vi "impulse.vi"() -> ()   [LabVIEW 2015]
uses:
  <vilib>/express/express analysis/Spectral/Block/exnSpectralBlock spectral measurements RMS poly.vi
  <vilib>/express/express analysis/Spectral/Block/exnSpectralBlock spectral measurements RMS WFM.vi
  <vilib>/express/express analysis/Spectral/XNode/ExpressSpectralMeasurementsBlockNode.xnode
panel:
  out "error out":errorcluster
  in  "error in":errorcluster
  in  "Stop Button":bool
  in  "Rate":dbl=4000.0
  in  "Averages":dbl=10.0
  in  "Time (sec)":dbl=0.2
  out "FFT":cluster{"f0":dbl, "df":dbl, "magnitude":dbl[]}(graph)={"f0"=0.0, "df"=5.0, "magnitude"=[-76.96384322517771, -76.42679486233023, -72.85666642341076, -71.38647319065812, -70.14662433053286, -67.52954782473027, -68.48400168826473, -72.39914045035815, -73.87927581141093, -76.83283155880913, -68.18744880683296, -68.4682142733081, -65.23066848529315, -69.27070672338077, -71.0175747468924, -73.06274814845091, -70.13008167063762, -76.36995304006233, -75.77281317706263, -75.55570327595308, -69.78822078992803, -68.74398541895071, -71.8694071583193, -64.49841394636594, -62.6804616224581, -66.92788976349084, -61.60831729458516, -62.28071166288875, -57.653094015959745, -53.22277642336562, -45.26642983314452, -34.38407325316543, -29.142428384242063, -32.91095376852357, -44.25910915056805, -53.18033994048258, -59.4769321245915, -61.072306867585986, -67.42925441188714, -66.84917435783197, -68.66575018363679, -69.7591404271292, -71.03152031159054, -70.9893803258124, -68.38199207817071, -72.00448948746491, -68.01256152070326, -67.9316604541294, -68.08904411886591, -67.99455524325555, -68.45174479754071, -67.30715293001177, -69.20448006996517, -67.5542171673227, -70.46036907543153, -67.58462190001059, -70.28521679448141, -68.2887848064451, -71.01143222397984, -67.6571419445792, -64.8548009674459, -63.820552592220196, -59.22957694885139, -52.5909165554164, -45.60812098925769, -42.002043104158304, -43.1903623164439, -49.22576249781181, -54.3780871023297, -57.86663523243824, -61.37809785909429, -65.05174356042342, -64.63930926360648, -64.11899085358468, -66.2159413011727, -68.93297817441363, -67.65564424572169, -72.9860971642846, -70.8799512804249, -74.08075178434568, -73.53297038665296, -74.1334014855353, -73.62832977107102, -74.71414022509782, -69.6031859659534, -70.21674262130918, -70.17200512340543, -68.8508491485637, -67.28457145151319, -67.18061516068467, -65.54873963096921, -65.0729025484959, -64.35822791542905, -61.6748482258688, -61.782563080853635, -63.04528441289746, -58.154907346835685, -54.71707233923819, -52.32393128109371, -53.81718862378017, -56.7098876504202, -62.68891050590184, -66.62682561685475, -66.83733759788919, -71.2450353090801, -65.65204670851749, -65.17581139718769, -68.16827380079054, -67.40143134206475, -67.11770285587087, -70.19719870933834, -67.87984510416211, -68.79990506319385, -71.59294042822327, -70.91779533548043, -71.37930707684605, -73.18467103419579, -74.5011236027276, -76.60216907463567, -76.36296374745734, -76.45992372880559, -73.34261139404917, -77.95153696406045, -72.05050193571411, -71.29187913220059, -69.62859338533406, -64.40675607726061, -63.35442870012269, -61.72236714640202, -57.662771066358744, -52.796942960053, -46.34620361215351, -42.96197942024599, -45.17513798727579, -51.64747739619454, -58.029749238153265, -63.58841604408845, -70.76172686722498, -74.0431297812586, -74.9889309405747, -72.52553568570184, -79.44586305416209, -75.57818400702382, -80.6207143763097, -75.45228631067108, -74.26272136812842, -77.05517432462732, -80.75333514371572, -74.95436340173164, -77.7343141563188, -75.08345145489872, -73.34506006774251, -77.47698539624334, -81.19713534940053, -76.00473310433264, -75.42901615687343, -78.20571496514997, -86.39258933247719, -79.06551886154028, -77.89189547590172, -76.14393205620179, -72.93536567376772, -67.13766563289994, -60.84765888264903, -51.58315520325594, -46.47566832056483, -48.54804136630699, -56.46988012444743, -64.11642116158627, -64.5786281646024, -68.2789885346105, -75.50097459432686, -71.83221105685784, -83.66782491984347, -75.27823026551795, -79.91546413793313, -84.70037150416685, -80.37298184889379, -90.1157689151875, -79.92871393538528, -84.83378559249539, -90.65780463744412, -81.34788679276531, -81.13427799763167, -86.04606910008829, -86.06641360780303, -78.28991024552357, -89.64816068193657, -80.8415647684923, -76.86141990488758, -83.5463763501563, -82.65373729606111, -73.75131007003918, -73.1974150846216, -73.1389997357267, -71.88763088714863, -68.92135534739391, -60.2018529106938, -55.89209342955029, -59.20342116383752, -66.40916834876512, -72.63324321776088, -75.30892178225696, -85.14599467373729, -82.6371796990402, -76.8616932072628, -78.73131182614961, -77.60434868224353, -78.05227652249873, -83.70865742856554, -82.55297700984232, -94.03545009272696, -80.044471309499, -81.33544305439534, -87.20188454329838, -98.67608701021186, -81.66188906785425, -91.03843676704793, -81.2031865773242, -78.37122122259265, -85.63224129946573, -80.83086428923929, -84.76759947185533, -86.76272267418442, -86.2432787532802, -74.50923605465248, -75.05979976616584, -73.29544535651468, -68.79120497441045, -63.791130306205986, -52.4284261430813, -46.359836741652884, -48.47279626546324, -57.63475431169838, -68.77762548022864, -66.49581278221342, -68.99764488031126, -80.55866874139923, -92.00918850330035, -83.88047913750569, -87.02579162228916, -82.09674572760248, -83.68654835147717, -104.51263565942185, -85.82853947797838, -89.43370352546552, -79.68190327152244, -94.73035123535304, -81.45037456045507, -81.8084869945688, -83.46509368403682, -88.81108803282159, -92.8086644359297, -83.58790453703016, -83.2136450944488, -88.51229855731462, -92.05735413219271, -90.02457676454648, -87.2517813101264, -87.28120307334017, -81.92442539538919, -76.43257493981947, -73.51313886097043, -63.25086201730103, -54.31781352775418, -54.244639260084725, -62.7932520240767, -69.76567406445712, -68.23203397736935, -65.11602803644264, -69.81065208507731, -79.09561936819793, -93.35790960218023, -91.00842555054459, -81.91127567754107, -82.80619456868445, -81.03736439222348, -86.8904445176983, -92.45913036981369, -90.26378282656839, -80.41232906278522, -86.34611608068853, -85.53962556031729, -84.17611136247531, -82.83916557111304, -81.39353257311132, -82.41185102059669, -93.90809308667906, -89.60421693224308, -88.73881675988, -88.68097298286662, -89.02865327589082, -81.84896452809127, -76.0251868961856, -92.52294540538264, -74.81196158037578, -74.79883036366476, -64.79374801683247, -62.61968008372651, -69.34007335638016, -74.49350463572966, -78.91626658507906, -76.60242821929597, -73.8397398347443, -76.89365702202115, -85.77212458607906, -92.01068000362652, -92.45268911423268, -84.90850285183336, -86.3157006646176, -83.9139294182518, -87.38676097510547, -80.45680693898265, -86.31794130868423, -85.71597308378712, -86.4651796575876, -83.69619571403283, -87.87844217547728, -88.05288102327424, -84.17388567859808, -85.3899832218231, -83.8854149022832, -92.31629119477367, -82.96936213243274, -90.84142527421787, -79.0415960446743, -75.19893969995199, -82.407681391743, -77.84498022849307, -68.97239189958741, -58.458869630375474, -54.298717457924646, -58.04807659734336, -66.64176322290302, -73.475869474644, -67.61018693803815, -67.60409308131246, -72.8458531358561, -82.83777471855413, -89.69423297549523, -83.74835563213936, -83.74557025458327, -85.9885542004791, -84.27652574443891, -82.48895125570638, -89.80178357196445, -87.41112039324227, -88.81410997820838, -85.93765535907339, -78.39101937805222, -80.6487164132958, -84.86455793235507, -90.58427007777658, -87.96735792934751, -85.77080994817338, -82.62355289779586, -94.85368124747853, -86.88270757865126, -84.08557415850237, -103.71835991722996, -81.4317418026578, -83.91842347605625, -86.60096717875804, -68.2069569784318, -61.555843858873246, -62.67891313799286, -68.5872453169184, -76.80705720169937, -64.40374534728049, -62.178896582762285, -66.80223049774496, -78.76625873591425, -80.33186795835033, -84.45597373359233, -91.94528099375434, -80.47827433656434, -80.19435355104328, -99.71603413141014, -83.10159194952354, -87.59893788907516, -86.53344535874828, -93.5292416047802, -86.46659686557426, -90.08228493067932, -83.59546583030911, -83.03139098879427, -89.30601507050662, -82.3822621204632, -84.80798276174946, -88.83824823006498, -78.73210732974867, -76.45438767337977, -79.87064358941596, -84.18025866857106, -85.89877761743617, -77.97963841715455, -84.7698939425612, -70.79328472827959, -70.717850793474, -76.01737083403677]}
  out "Impulse":waveform(dbl)(graph)={"t0"=timestamp(0 s since 1904-01-01), "dt"=0.00025, "Y"=array[800 elements]}
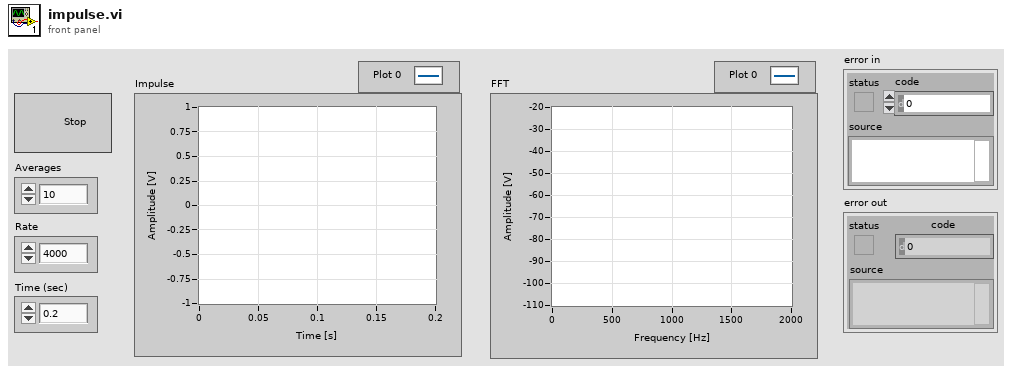
[diagram p1: front panel]
types:
  T1 = cluster{"averaging mode":u16, "weighting mode":u16, "number of averages":u32}
  T2 = cluster{"dB On (F)":bool, "unwrap phase (F)":bool, "convert to degree (F)":bool}
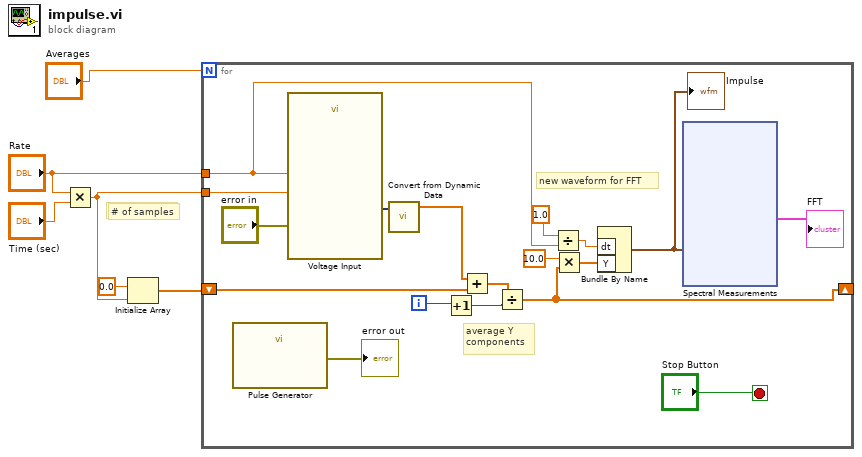
[diagram p0: block diagram]
diagram:
  # "# of samples"
  # "# of samples"
  n1 = Multiply(x="Rate", y="Time (sec)") -> (x*y=w3:dbl)
  n2 = Initialize Array(0.0 ("element"), w3) -> (w1:dbl[])
  n3 = for {
    N: "Averages" -> [_]
    tunnel: w3 -> [w24]
    tunnel: "Rate" -> [w8]
    shift-right: [w16] -> _
    shift-left: w1 -> [w21]
    i -> [w13]
    stop <- "Stop Button" stop-if-true
    # "new waveform for FFT"
    # "average Y \ncomponents"
    n4 = call "Pulse Generator"() -> ("error out"=→"error out":errorcluster)  [unwired: 18 in, 1 out]
    n5 = call "Voltage Input"("rate"=w8, "number of samples"=w24, "error in"="error in") -> ("data"=w22:dynamicdata)  [unwired: 14 in, 2 out]
    n6 = call "Convert from Dynamic Data"("Dynamic Data Type"=w22) -> ("Array"=w11:dbl[])  [unwired: 3 in]
    n7 = Increment(x=w13) -> (x+1=w12:i32)
    n8 = Add(x=w11, y=w21) -> (x+y=w20:dbl[])
    n9 = Divide(x=w20, y=w12) -> (x/y=w16:dbl[])
    n10 = Divide(x=1.0, y=w8) -> (x/y=w7:dbl)
    n11 = Multiply(x=10.0 ("y"), y=w16) -> (x*y=w10:dbl[])
    n12 = Bundle By Name("dt"=w7, "Y"=w10) -> (w18:waveform(dbl))  [unwired: 1 in]
    "Impulse" <- w18
    n13 = xnode "Spectral Measurements"("Signals"=w18) -> ("FFT - (RMS)"=→"FFT":cluster{"f0":dbl, "df":dbl, "magnitude":dbl[]})  [unwired: 1 in, 2 out]
  }
